vi "EstimateGCost.vi"(9 "Nó pai":dbl[](array[numeric]), 10 "Nó atual":dbl[](array[numeric]), 11 "GridParameter":dbl) -> (2 "G_Cost":dbl)   [LabVIEW 2016]
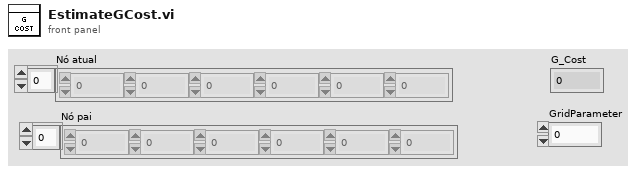
[diagram p1: front panel]
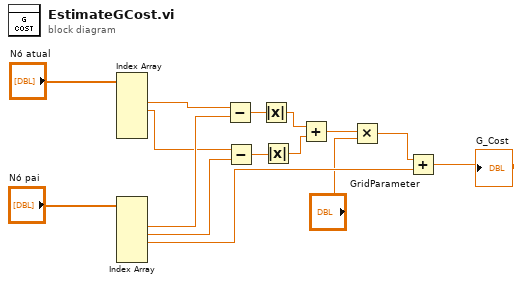
[diagram p0: block diagram]
diagram:
  n1 = Index Array(array="Nó atual") -> (element #2=w12:dbl, element #3=w9:dbl)  [unwired: 6 in, 4 out]
  n2 = Index Array(array="Nó pai") -> (element #2=w11:dbl, element #3=w8:dbl, element #4=w13:dbl)  [unwired: 6 in, 3 out]
  n3 = Subtract(x=w12, y=w11) -> (x-y=w10:dbl)
  n4 = Subtract(x=w9, y=w8) -> (x-y=w7:dbl)
  n5 = Absolute Value(x=w10) -> (abs(x)=w5:dbl)
  n6 = Absolute Value(x=w7) -> (abs(x)=w6:dbl)
  n7 = Add(x=w5, y=w6) -> (x+y=w3:dbl)
  n8 = Multiply(x=w3, y="GridParameter") -> (x*y=w2:dbl)
  n9 = Add(x=w2, y=w13) -> (x+y=→"G_Cost":dbl)
